vi "Do Failure Action.vi"(8 "error in (no error)":errorcluster, 11 "Assert Message in":T1) -> (0 "error out":errorcluster)   [LabVIEW 2017, in "Assert API Components.lvlib" / "Log Assert Core.lvlib"]
uses:
  Log Assert Core.lvlib
  Message Data.ctl
  Failure Actions.ctl
  Failure Actions/Abort Application/Abort Application.lvclass
  C:/Users/ukhornp/Documents/Work/Projects/actor_assert_api/Core/Assert API Components/Log Assert Core Components/Failure Actions/Fail Action Base.lvclass
  Failure Actions/Log To File/Log To File.lvclass
  Failure Actions/Fail Action Base.lvclass
  Failure Actions/Pause Application/Pause Application.lvclass
  Assert API Components.lvlib
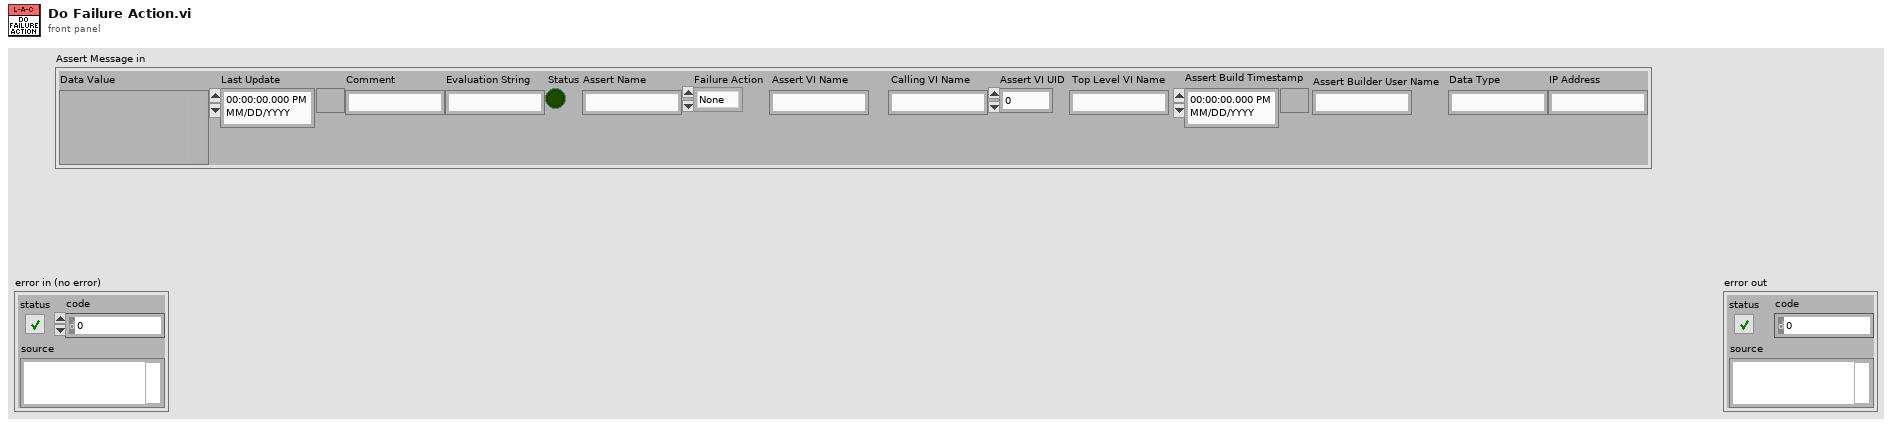
[diagram p1: front panel]
types:
  T1 = typedef "Assert API Components.lvlib/Message Data.ctl" = cluster{"Data Value":variant, "Last Update":timestamp, "Comment":string, "Evaluation String":string, "Status":bool, "Assert Name":string, "Failure Action":T2, "Assert VI Name":string, "Calling VI Name":string, "Assert VI UID":i32, "Top Level VI Name":string, "Assert Build Timestamp":timestamp, "Assert Builder User Name":string, "Data Type":string, "IP Address":string}
  T2 = typedef "Assert API Components.lvlib/Failure Actions.ctl" = enum16{"None", "Log To File", "Pause Execution", "Abort Execution"}
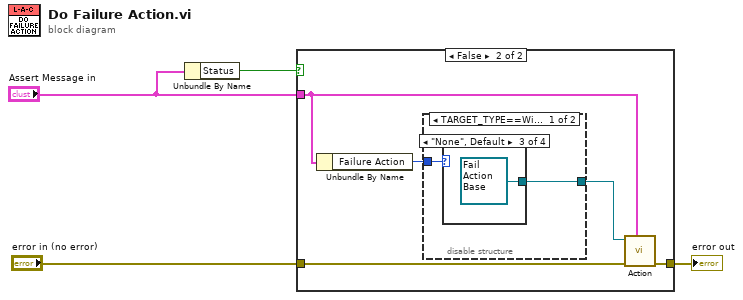
[diagram p0: block diagram]
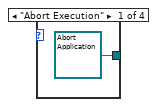
[diagram p3: hidden frame]
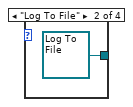
[diagram p4: hidden frame]
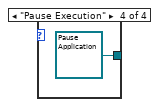
[diagram p5: hidden frame]
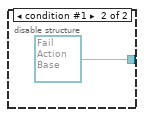
[diagram p6: hidden frame]
diagram:
  n1 = Unbundle By Name("Assert Message in") -> ("Status"=w1:bool)
  n2 = case shown="False" w1 {
    tunnel: "error in (no error)" -> [w5 w10]
    tunnel: "Assert Message in" -> [_ w7]
    tunnel: [w5 w8] -> w4
    frame True {
      # "Assert passed - no action"
    }
    frame False {
      n3 = Unbundle By Name(w7) -> ("Failure Action"=w6:T2)
      n4 = disable-structure shown="TARGET_TYPE==Windows" {
        disable-tunnel: w6 -> [w12 _]
        disable-tunnel: [w11 refnum<class "Fail Action Base.lvclass"> refnum ("Assert API Components.lvlib:Log Assert Core.lvlib:Fail Action Base.lvclass")] -> w9
        frame condition #0 (active) {
          n5 = case shown="\"None\", Default" w12 {
            tunnel: [refnum<class "Abort Application.lvclass"> refnum ("Assert API Components.lvlib:Log Assert Core.lvlib:Abort Application.lvclass") refnum<class "Log To File.lvclass"> refnum ("Assert API Components.lvlib:Log Assert Core.lvlib:Log To File.lvclass") refnum<class "Fail Action Base.lvclass"> refnum ("Assert API Components.lvlib:Log Assert Core.lvlib:Fail Action Base.lvclass") refnum<class "Pause Application.lvclass"> refnum ("Assert API Components.lvlib:Log Assert Core.lvlib:Pause Application.lvclass")] -> w11
            frame "Abort Execution" {
            }
            frame "Log To File" {
            }
            frame "None", Default {
            }
            frame "Pause Execution" {
            }
          }
        }
        frame condition #1 {
        }
      }
      n6 = call-dynamic "Action.vi"("Assert Message"=w7, "error in (no error)"=w10, "Fail Action Base in"=w9) -> ("error out"=w8:errorcluster)  [unwired: 8 in]
    }
  }
  "error out" <- w4
